vi "nominal ingest job status.vi"(8 "error in (no error)":errorcluster, 10 "out_status":i32, 11 "job":i32) -> (0 "error out":errorcluster, 2 "out_status out":i32, 3 "function return":i32)   [LabVIEW 2020, in "client.lvlib"]
doc: "int32_t nominal_ingest_job_status(int32_t job, int32_t *out_status);"
uses:
  client.lvlib
  bin/nominalClient_64.dll
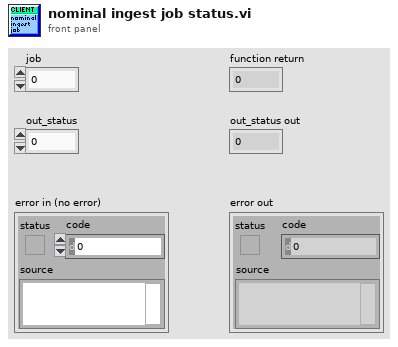
[diagram p1: front panel]
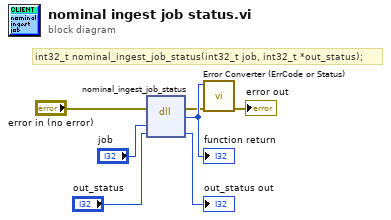
[diagram p0: block diagram]
diagram:
  # "int32_t nominal_ingest_job_status(int32_t job, int32_t *out_status);"
  n1 = dll-call lib="C:/code/labview-client-rs/lv_src/bin/nominalClient_*.*" fn="nominal_ingest_job_status"(error in="error in (no error)", "job"="job", "out_status"="out_status") -> (error out=w2:errorcluster, w7:i32, "out_status"=→"out_status out":i32)  [unwired: 3 in, 1 out]
  "function return" <- w7
  n2 = call "Error Converter (ErrCode or Status).vi"("error in (no error)"=w2, "error code"=w7) -> ("error out"=→"error out":errorcluster)  [unwired: 9 in]
